vi "DriveStraight.vi"(10 "Distance":dbl, 11 "Speed":dbl) -> (2 "At Distance":bool)   [LabVIEW 2011]
panel:
  in  "Encoder Gain - Slow":dbl=0.005
  in  "Encoder Gain - Fast":dbl=0.0085
  in  "Sensitivity":dbl=1.0
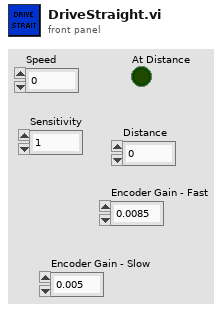
[diagram p1: front panel]
types:
  T1 = cluster{"Speed Right":dbl, "Distance Right":dbl, "Speed Left":dbl, "Distance Left":dbl}
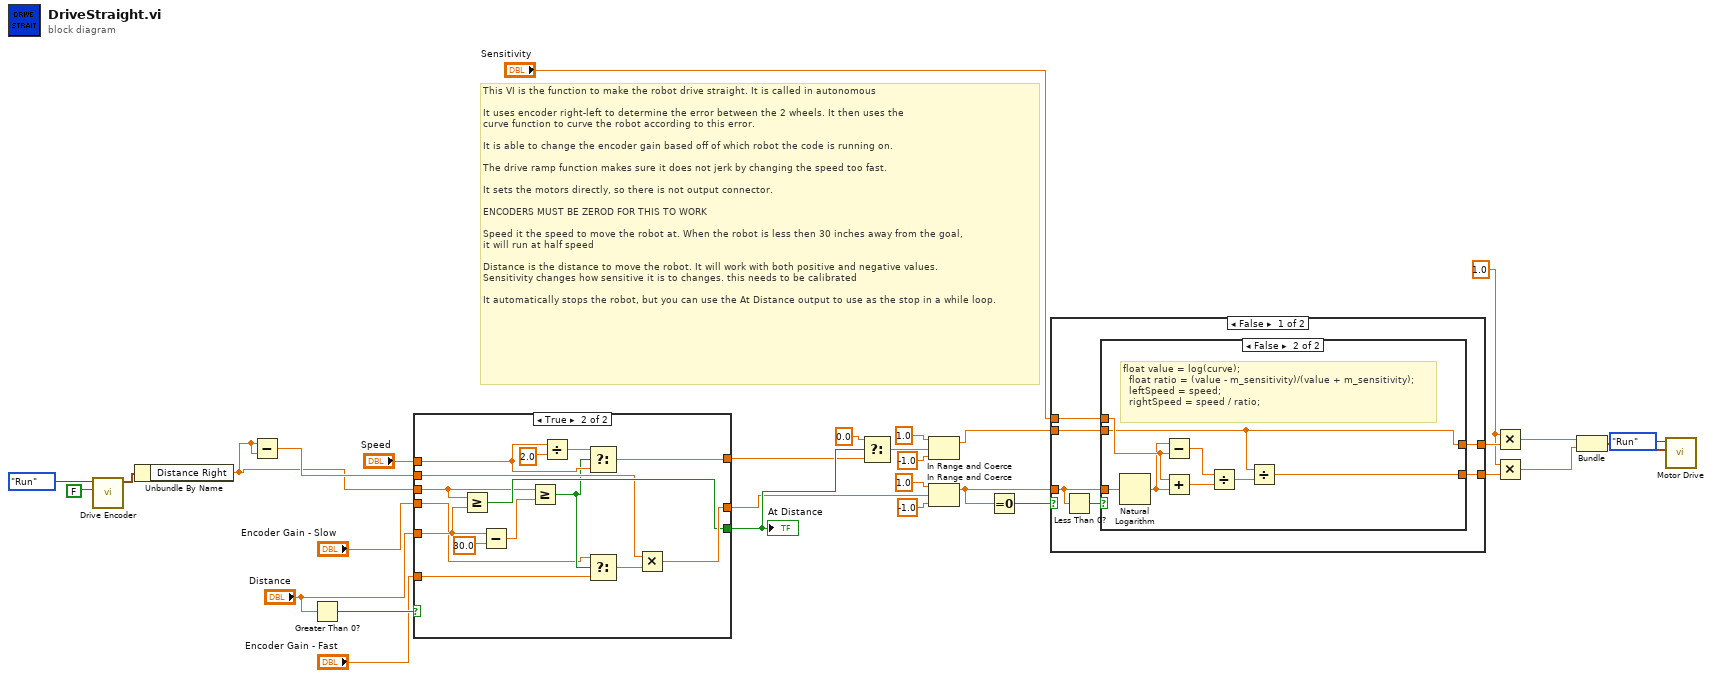
[diagram p0: block diagram]
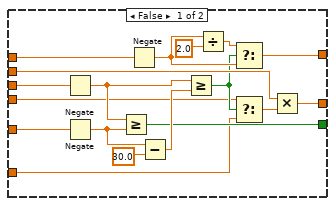
[diagram p2: hidden frame]
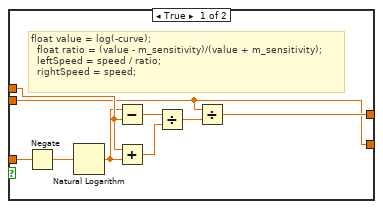
[diagram p3: hidden frame]
diagram:
  w21 = 1.0
  # "This VI is the function to make the robot drive straight. It is called in autonomous\n\nIt uses encoder right-left to determine the error between the 2 wheels. It then uses the\ncurve function to curve the robot according to this error.\n\nIt is able to change the encoder gain based off of which robot the code is running on.\n\nThe drive ramp function makes sure it does not jerk by changing the speed too fast.\n\nIt sets the motors directly, so there is not output connector.\n\nENCODERS MUST BE ZEROD FOR THIS TO WORK\n\nSpeed it the speed to move the robot at. When the robot is less then 30 inches away from the goal,\nit will run at half speed\n\nDistance is the distance to move the robot. It will work with both positive and negative values.\nSensitivity changes how sensitive it is to changes. this needs to be calibrated\n\nIt automatically stops the robot, but you can use the At Distance output to use as the stop in a while loop."
  n1 = call "Drive Encoder.vi"("Reset"=FALSE, "Enum"=enum16{"Init", "Run", "End"}."Run") -> ("Encoder Values"=w6:T1)  [unwired: 9 in]
  n2 = Unbundle By Name(w6) -> ("Distance Right"=w2:dbl)
  n3 = Subtract(x=w2, y=w2) -> (x-y=w5:dbl)
  n4 = Greater Than 0?(x="Distance") -> (x > 0?=w20:bool)
  n5 = case shown="True" w20 {
    tunnel: [w48 w63] -> w13
    tunnel: w2 -> [w39 w61]
    tunnel: "Distance" -> [w40 w59]
    tunnel: [w43 w62] -> w17
    tunnel: "Speed" -> [w37 w55]
    tunnel: [w42 w54] -> w15
    tunnel: w5 -> [w35 w53]
    tunnel: "Encoder Gain - Fast" -> [w32 w50]
    tunnel: "Encoder Gain - Slow" -> [w33 w49]
    frame False {
      n6 = Negate(x=w39) -> (-x=w38:dbl)
      n7 = Negate(x=w40) -> (-x=w41:dbl)
      n8 = Greater Or Equal?(x=w38, y=w41) -> (x >= y?=w43:bool)
      n9 = Negate(x=w37) -> (-x=w36:dbl)
      n10 = Subtract(x=w41, y=30.0) -> (x-y=w44:dbl)
      n11 = Greater Or Equal?(x=w38, y=w44) -> (x >= y?=w34:bool)
      n12 = Divide(x=w36, y=2.0) -> (x/y=w47:dbl)
      n13 = Select(t=w47, s=w34, f=w36) -> (s? t:f=w42:dbl)
      n14 = Select(t=w33, s=w34, f=w32) -> (s? t:f=w31:dbl)
      n15 = Multiply(x=w35, y=w31) -> (x*y=w48:dbl)
    }
    frame True {
      n16 = Greater Or Equal?(x=w61, y=w59) -> (x >= y?=w62:bool)
      n17 = Subtract(x=w59, y=30.0) -> (x-y=w60:dbl)
      n18 = Greater Or Equal?(x=w61, y=w60) -> (x >= y?=w52:bool)
      n19 = Divide(x=w55, y=2.0) -> (x/y=w56:dbl)
      n20 = Select(t=w56, s=w52, f=w55) -> (s? t:f=w54:dbl)
      n21 = Select(t=w49, s=w52, f=w50) -> (s? t:f=w51:dbl)
      n22 = Multiply(x=w53, y=w51) -> (x*y=w63:dbl)
    }
  }
  "At Distance" <- w17
  n23 = Select(t=0.0, s=w17, f=w15) -> (s? t:f=w14:dbl)
  n24 = In Range and Coerce(upper limit=1.0, x=w14, lower limit=-1.0) -> (coerced(x)=w4:dbl)  [unwired: 1 out]
  n25 = In Range and Coerce(upper limit=1.0, x=w13, lower limit=-1.0) -> (coerced(x)=w23:dbl)  [unwired: 1 out]
  n26 = Equal To 0?(x=w23) -> (x = 0?=w30:bool)
  n27 = case shown="False" w30 {
    tunnel: w4 -> [w68 w87]
    tunnel: [w65 w87] -> w29
    tunnel: [w64 w87] -> w28
    tunnel: w23 -> [w67 _]
    tunnel: "Sensitivity" -> [w66 _]
    frame False {
      n28 = Less Than 0?(x=w67) -> (x < 0?=w69:bool)
      n29 = case shown="False" w69 {
        tunnel: w66 -> [w75 w86]
        tunnel: w67 -> [w76 w85]
        tunnel: w68 -> [w71 w81]
        tunnel: [w72 w81] -> w65
        tunnel: [w71 w79] -> w64
        frame True {
          # "float value = log(-curve);\n\t\tfloat ratio = (value - m_sensitivity)/(value + m_sensitivity);\n\t\tleftSpeed = speed / ratio;\n\t\trightSpeed = speed;"
          n30 = Negate(x=w76) -> (-x=w74:dbl)
          n31 = Natural Logarithm(1:w74) -> (0:w70:dbl)
          n32 = Subtract(x=w70, y=w75) -> (x-y=w78:dbl)
          n33 = Add(x=w75, y=w70) -> (x+y=w77:dbl)
          n34 = Divide(x=w78, y=w77) -> (x/y=w73:dbl)
          n35 = Divide(x=w71, y=w73) -> (x/y=w72:dbl)
        }
        frame False {
          # "float value = log(curve);\n\t\tfloat ratio = (value - m_sensitivity)/(value + m_sensitivity);\n\t\tleftSpeed = speed;\n\t\trightSpeed = speed / ratio;"
          n36 = Natural Logarithm(1:w85) -> (0:w84:dbl)
          n37 = Subtract(x=w84, y=w86) -> (x-y=w83:dbl)
          n38 = Add(x=w86, y=w84) -> (x+y=w82:dbl)
          n39 = Divide(x=w83, y=w82) -> (x/y=w80:dbl)
          n40 = Divide(x=w81, y=w80) -> (x/y=w79:dbl)
        }
      }
    }
    frame True {
    }
  }
  n41 = Multiply(x=w21, y=w29) -> (x*y=w12:dbl)
  n42 = Multiply(x=w21, y=w28) -> (x*y=w11:dbl)
  n43 = Bundle(w12, w11) -> (w3:cluster{dbl, dbl})  [unwired: 1 out]
  n44 = call "Motor Drive.vi"("Motor Input"=w3, "Enum"=enum16{"Init", "Run", "SetBrakeCoast", "End"}."Run") -> ()  [unwired: 10 in]
